vi "Host-OrderBook-TestHarness.vi"() -> ()   [LabVIEW 2016]
uses:
  <vilib>/rvi/interface/RandomDataEmulation/nirviRandomDataOpen.vi
  <vilib>/rvi/interface/RandomDataEmulation/nirviRandomDataDMAMethods.vi
  <vilib>/rvi/interface/RandomDataEmulation/nirviRandomDataClose.vi
  <vilib>/rvi/interface/nirviOpenFPGA/nirviOpenFPGA.xnode
  OrderBook-TestHarness-Typedef.ctl
  Fpga/Tests/Fpga-OrderBook-TestHarness.vi
  <vilib>/rvi/interface/nirviMethod/nirviMethod.xnode
  <vilib>/rvi/interface/nirviCloseFPGA/nirviCloseFPGA.xnode
panel:
  out "OrderBook Array":T1(array[cluster])
  in  "OrderBook-Commands":T2(array[cluster])=[{"Operation"=enum."AddOrder", "Cluster"={"Side"=enum."Buy", "OrderRefNum"=103, "Price"=1012500, "Shares"=100}}, {"Operation"=enum."AddOrder", "Cluster"={"Side"=enum."Buy", "OrderRefNum"=110, "Price"=1012400, "Shares"=200}}, {"Operation"=enum."AddOrder", "Cluster"={"Side"=enum."Buy", "OrderRefNum"=120, "Price"=1012600, "Shares"=300}}, {"Operation"=enum."GetAll", "Cluster"={"Side"=enum."Sell", "OrderRefNum"=0, "Price"=0, "Shares"=0}}]
  out "error out":errorcluster
  in  "error in":errorcluster
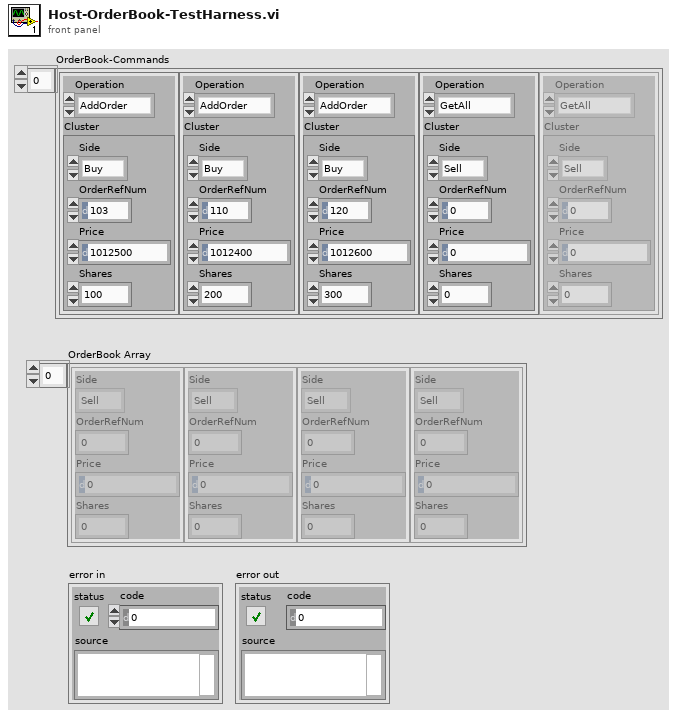
[diagram p1: front panel]
types:
  T1 = cluster{"Side":enum16{"Sell", "Buy"}, "OrderRefNum":u64, "Price":u32, "Shares":u32}[]
  T2 = cluster{"Operation":enum16{"Noop", "GetAll", "AddOrder", "DeleteOrder"}, "Cluster":cluster{"Side":enum16{"Sell", "Buy"}, "OrderRefNum":u64, "Price":u32, "Shares":u32}}[]
  T3 = typedef "OrderBook-TestHarness-Typedef.ctl" = refnum<k20>
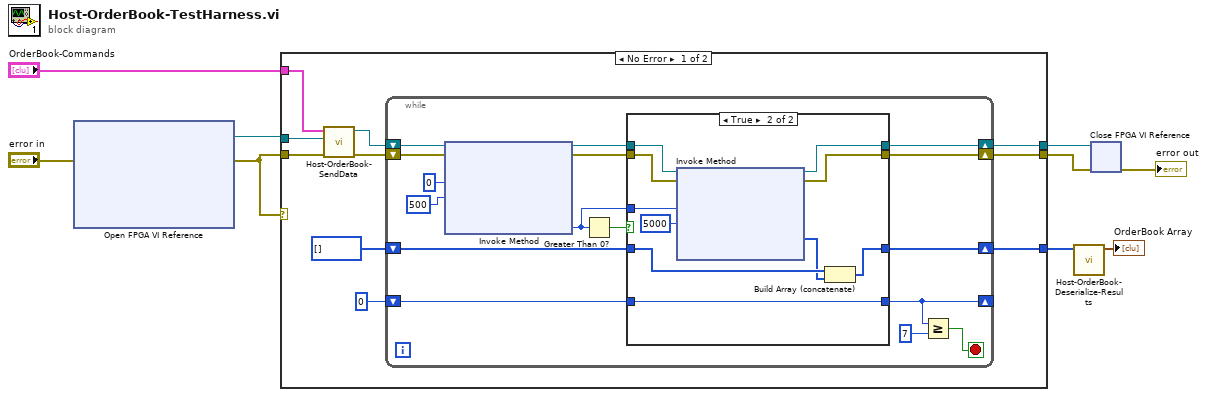
[diagram p0: block diagram]
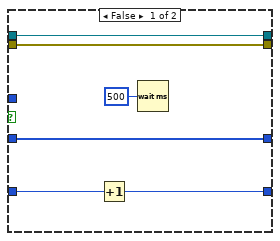
[diagram p2: hidden frame]
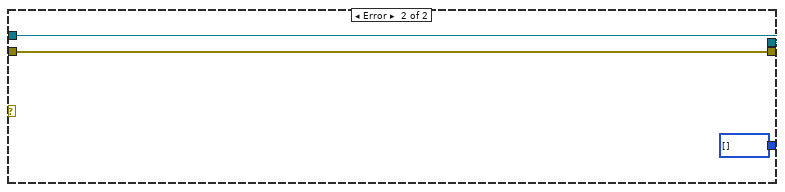
[diagram p3: hidden frame]
diagram:
  n1 = xnode "Open FPGA VI Reference"("error in"="error in") -> ("FPGA VI Reference Out"=w9:T3, "error out"=w6:errorcluster)  [unwired: 1 in]
  n2 = case shown="No Error" w6 {
    tunnel: w9 -> [w11 w53]
    tunnel: [w19 w54] -> w3
    tunnel: w6 -> [w12 w54]
    tunnel: [w18 w53] -> w1
    tunnel: [w15 u64[] [] ("Data 2")] -> w4
    tunnel: "OrderBook-Commands" -> [w14 _]
    frame No Error {
      n3 = call "Host-OrderBook-SendData.vi"("error in"=w12, "FPGA VI Reference in"=w11, "OrderBook-Commands"=w14) -> ("error out"=w13:errorcluster, "FPGA VI Reference out"=w10:T3)  [unwired: 7 in]
      n4 = while {
        shift-right: [w24] -> w15
        shift-left: u64[] [] ("Data 2") -> [w25]
        shift-right: [w27] -> w18
        shift-left: w10 -> [w35]
        shift-right: [w26] -> w19
        shift-left: w13 -> [w28]
        shift-right: [w22] -> _
        shift-left: 0 -> [w23]
        stop <- w20 stop-if-true
        n5 = xnode "Invoke Method"("FPGA VI Reference In"=w35, "error in"=w28, "Number of Elements"=u32 0, "Timeout (ms)"=500) -> ("FPGA VI Reference Out"=w30:T3, "error out"=w29:errorcluster, "Elements Remaining"=w31:u32)  [unwired: 1 out]
        n6 = Greater Than 0?(x=w31) -> (x > 0?=w32:bool)
        n7 = case shown="True" w32 {
          tunnel: w31 -> [_ w51]
          tunnel: w30 -> [w41 w49]
          tunnel: w29 -> [w40 w48]
          tunnel: [w41 w47] -> w27
          tunnel: [w40 w46] -> w26
          tunnel: w25 -> [w39 w45]
          tunnel: [w39 w43] -> w24
          tunnel: [w37 w42] -> w22
          tunnel: w23 -> [w38 w42]
          frame False {
            n8 = Increment(x=w38) -> (x+1=w37:i32)
            n9 = Wait (ms)(milliseconds to wait=u32 500) -> ()  [unwired: 1 out]
          }
          frame True {
            n10 = xnode "Invoke Method"("FPGA VI Reference In"=w49, "error in"=w48, "Number of Elements"=w51, "Timeout (ms)"=5000) -> ("FPGA VI Reference Out"=w47:T3, "error out"=w46:errorcluster, "Data"=w44:u64[])  [unwired: 1 out]
            n11 = Build Array (concatenate)(w45, w44) -> (w43:u64[])
          }
        }
        n12 = Greater Or Equal?(x=w22, y=7) -> (x >= y?=w20:bool)
      }
    }
    frame Error {
    }
  }
  n13 = call "Host-OrderBook-Deserialize-Results.vi"("Data in"=w4) -> ("OrderBook Array"=→"OrderBook Array":T1)  [unwired: 10 in]
  n14 = xnode "Close FPGA VI Reference"("FPGA VI Reference In"=w1, "error in"=w3) -> ("error out"=→"error out":errorcluster)
